vi "collsions_at_different_pressures.vi"() -> ()   [LabVIEW 2019]
uses:
  <instrlib>/niScope/Controls/niScope vertical coupling.ctl
  <instrlib>/niScope/Controls/niScope trigger source.ctl
  <instrlib>/niScope/Controls/niScope trigger coupling.ctl
  <instrlib>/niScope/Controls/niScope trigger slope.ctl
  <vilib>/Waveform/WDTFileIO.llb/Export Waveform To Spreadsheet File.vi
  <vilib>/Analysis/NI_AALBase.lvlib
panel:
  in  "Lower bound":dbl=4e-06
  in  "Step size":dbl=5e-07
  in  "Upper bound":dbl=5e-05
  in  "Channel":u16(ring) items=["1", "2"]
  in  "Eqilibration time / s":u32
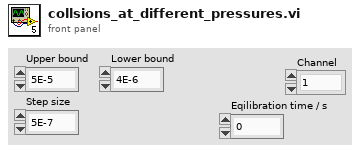
[diagram p1: front panel]
types:
  T1 = typedef "niScope vertical coupling.ctl" = i32
  T2 = typedef "niScope trigger source.ctl" = string
  T3 = typedef "niScope trigger coupling.ctl" = u16
  T4 = typedef "niScope trigger slope.ctl" = i32
  T5 = cluster{"C2 vertical offset":dbl, "C2 vertical range":dbl, "C2 probe attenuation":dbl, "C2 vertical coupling":T1, "C2 maximum input frequency":dbl, "C2 input impedance":u32, "C2 enabled":bool, "C1 input impedance":u32, "C1 maximum input frequency":dbl, "C1 enabled":bool, "C1 vertical offset":dbl, "C1 vertical range":dbl, "C1 probe attenuation":dbl, "C1 vertical coupling":T1, "Samples":i64, "tmax (\\mu s) ":dbl, "Trigger source":T2, "Trigger coupling":T3, "Trigger level":dbl, "Trigger slope":T4, "Trigger delay":dbl, "Enforce realtime":bool, "Aquisition Frequency / Hz":dbl, "Aqusition Time / ms":u32, "Scope Channel":refnum<k15>}
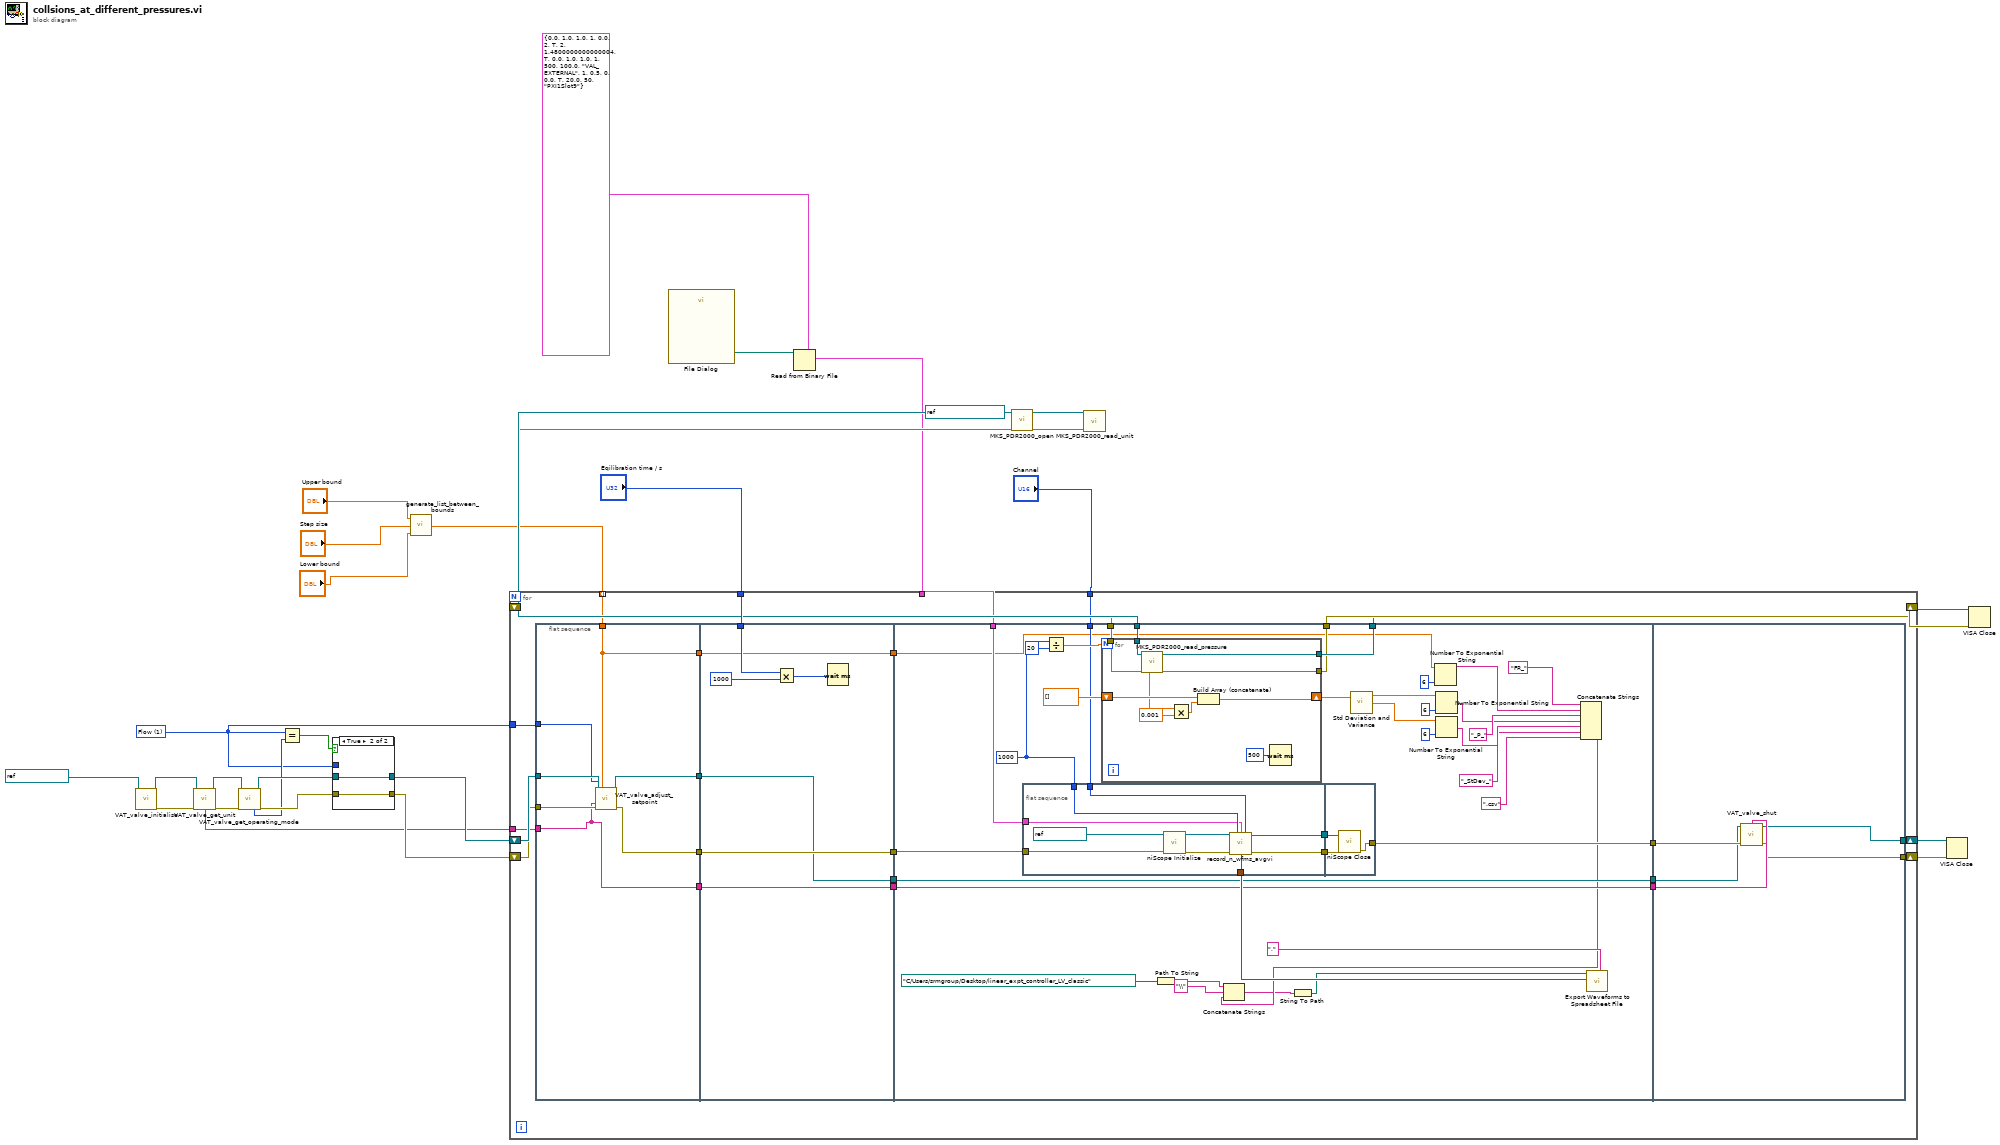
[diagram p0: block diagram]
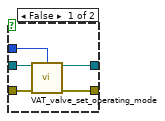
[diagram p2: hidden frame]
diagram:
  w19 = u16 1 items=["Pressure", "Flow", "Stop"] ("Operating Mode")
  n1 = call "VAT_valve_initialise.vi"("VAT Valve COM port"=refnum<visa-resource-name> "VAT_valve") -> ("VAT Valve COM port out"=w30:refnum<visa-resource-name>, "error out"=w29:errorcluster)  [unwired: 7 in, 6 out]
  n2 = call "VAT_valve_get_unit.vi"("VAT Valve COM port"=w30, "error in (no error)"=w29) -> ("VAT Valve COM port out"=w28:refnum<visa-resource-name>, "Unit"=w20:string, "error out"=w27:errorcluster)  [unwired: 11 in]
  n3 = call "VAT_valve_get_operating_mode.vi"("VAT Valve COM port"=w28, "error in (no error)"=w27) -> ("VAT Valve COM port out"=w26:refnum<visa-resource-name>, "Operating Mode"=w23:u16, "error out"=w25:errorcluster)  [unwired: 10 in, 1 out]
  n4 = Equal?(x=w19, y=w23) -> (x = y?=w24:bool)
  n5 = case shown="True" w24 {
    tunnel: w26 -> [w36 w38]
    tunnel: w25 -> [w35 w37]
    tunnel: [w34 w38] -> w22
    tunnel: [w33 w37] -> w21
    tunnel: w19 -> [w32 _]
    frame False {
      n6 = call "VAT_valve_set_operating_mode.vi"("VAT Valve COM port"=w36, "Operating Mode"=w32, "error in (no error)"=w35) -> ("VAT Valve COM port out"=w34:refnum<visa-resource-name>, "error out"=w33:errorcluster)  [unwired: 11 in]
    }
    frame True {
    }
  }
  n7 = call "generate_list_between_bounds.vi"("Upper bound"="Upper bound", "Step size"="Step size", "Lower bound"="Lower bound") -> ("Array"=w1:dbl[])  [unwired: 2 in]
  n8 = call "File Dialog"() -> ("selected path"=w9:path)  [unwired: 12 in, 3 out]
  n9 = Read from Binary File(5:T5 {"C2 vertical offset"=0.0, "C2 vertical range"=1.0, "C2 probe attenuation"=1.0, "C2 vertical coupling"=1, "C2 maximum input frequency"=0.0, "C2 input impedance"=2, "C2 enabled"=TRUE, "C1 input impedance"=2, "C1 maximum input frequency"=1.4800000000000004, "C1 enabled"=TRUE, "C1 vertical offset"=0.0, "C1 vertical range"=1.0, "C1 probe attenuation"=1.0, "C1 vertical coupling"=1, "Samples"=500, "tmax (\\mu s) "=100.0, "Trigger source"="VAL_EXTERNAL", "Trigger coupling"=1, "Trigger level"=0.5, "Trigger slope"=0, "Trigger delay"=0.0, "Enforce realtime"=TRUE, "Aquisition Frequency / Hz"=20.0, "Aqusition Time / ms"=50, "Scope Channel"="PXI1Slot9"} ("Cluster"), 11:w9) -> (2:w8:T5)  [unwired: 4 in, 3 out]
  n10 = call "MKS_PDR2000_open.vi"("PDR2000 COM port"=refnum<visa-resource-name> "PDR_2000") -> ("error out"=w15:errorcluster, "PDR2000 COM port out"=w16:refnum<visa-resource-name>)  [unwired: 9 in]
  n11 = call "MKS_PDR2000_read_unit.vi"("PDR2000 COM port"=w16, "error in (no error)"=w15) -> ("PDR2000 COM port out"=w14:refnum<visa-resource-name>, "error out"=w13:errorcluster)  [unwired: 11 in, 1 out]
  n12 = for {
    tunnel: w20 -> [w50]
    tunnel: w19 -> [w49]
    tunnel: "Eqilibration time / s" -> [w48]
    tunnel: w8 -> [w43]
    tunnel: "Channel" -> [w40]
    shift-right: [w42] -> w7
    shift-left: w22 -> [w52]
    shift-right: [w41] -> w6
    shift-left: w21 -> [w51]
    shift-right: [w44] -> w11
    shift-left: w14 -> [w47]
    shift-right: [w45] -> w12
    shift-left: w13 -> [w46]
    tunnel: w1 -> [w39] mode=indexing
    n13 = flat-sequence {
      tunnel: w52 -> [w70]
      tunnel: w51 -> [w69]
      tunnel: w50 -> [w65]
      tunnel: w39 -> [w64]
      tunnel: w49 -> [w68]
      tunnel: [w67] -> w63
      tunnel: [w66] -> w62
      tunnel: [w65] -> w61
      tunnel: [w64] -> w60
      tunnel: w48 -> [w76]
      tunnel: [w74] -> w59
      tunnel: w63 -> [w74]
      tunnel: [w73] -> w58
      tunnel: w62 -> [w73]
      tunnel: w61 -> [w72]
      tunnel: [w72] -> w57
      tunnel: [w71] -> w56
      tunnel: w60 -> [w71]
      tunnel: w47 -> [w115]
      tunnel: w46 -> [w114]
      tunnel: [w105] -> w45
      tunnel: [w113] -> w44
      tunnel: w59 -> [w111]
      tunnel: [w101] -> w55
      tunnel: w58 -> [w100]
      tunnel: [w100] -> w54
      tunnel: w43 -> [w99]
      tunnel: w57 -> [w98]
      tunnel: [w98] -> w53
      tunnel: w40 -> [w97]
      tunnel: w56 -> [w88]
      tunnel: w55 -> [w143]
      tunnel: w54 -> [w142]
      tunnel: w53 -> [w141]
      tunnel: [w140] -> w42
      tunnel: [w139] -> w41
      frame #0 {
        n14 = call "VAT_valve_adjust_setpoint.vi"("VAT Valve COM port"=w70, "Flow"=w64, "Operating Mode"=w68, "Unit"=w65, "error in (no error)"=w69) -> ("VAT Valve COM port out"=w66:refnum<visa-resource-name>, "error out"=w67:errorcluster)  [unwired: 9 in]
      }
      frame #1 {
        n15 = Multiply(x=w76, y=u32 1000 ("milliseconds to wait")) -> (x*y=w75:u32)
        n16 = Wait (ms)(milliseconds to wait=w75) -> ()  [unwired: 1 out]
      }
      frame #2 {
        w107 = 1000 ("Number of Sweeps")
        n17 = flat-sequence {
          tunnel: w111 -> [w132]
          tunnel: [w131] -> w110
          tunnel: [w130] -> w109
          tunnel: w107 -> [w129]
          tunnel: [w128] -> w102
          tunnel: w99 -> [w127]
          tunnel: w97 -> [w126]
          tunnel: w110 -> [w138]
          tunnel: w109 -> [w137]
          tunnel: [w136] -> w101
          frame #0 {
            n18 = call <instrlib>:"niScope Initialize.vi"("resource name"=refnum<k15> "PXI1Slot9" ("instrument handle"), "error in"=w132) -> ("instrument handle"=w135:refnum<k15>, "error out"=w134:errorcluster)  [unwired: 12 in]
            n19 = call "record_n_wfms_avgvi.vi"("instrument handle"=w135, "Number of Sweeps"=w129, "Scope Config Data"=w127, "Channel"=w126, "Error in (no error)"=w134) -> ("instrument handle out"=w131:refnum<k15>, "Waveform"=w128:waveform(dbl), "Error out"=w130:errorcluster)  [unwired: 8 in]
          }
          frame #1 {
            n20 = call <instrlib>:"niScope Close.vi"("instrument handle"=w138, "error in"=w137) -> ("error out"=w136:errorcluster)  [unwired: 13 in]
          }
        }
        n21 = Divide(x=w107, y=20) -> (x/y=w108:dbl)
        n22 = for {
          N: w108 -> [_]
          tunnel: w115 -> [w125]
          tunnel: w114 -> [w124]
          tunnel: [w123] -> w113
          tunnel: [w122] -> w105
          shift-right: [w120] -> w104
          shift-left: dbl[] [] -> [w121]
          n23 = call "MKS_PDR2000_read_pressure.vi"("error in (no error)"=w124, "PDR2000 COM port"=w125) -> ("error out"=w122:errorcluster, "PDR2000 COM port out"=w123:refnum<visa-resource-name>, "Channel 1 Pressure"=w118:dbl)  [unwired: 6 in, 1 out]
          n24 = Multiply(x=w118, y=0.001) -> (x*y=w119:dbl)
          n25 = Build Array (concatenate)(w121, w119) -> (w120:dbl[])
          n26 = Wait (ms)(milliseconds to wait=u32 500) -> ()  [unwired: 1 out]
        }
        n27 = Path To String(path=path "C:/Users/srmgroup/Desktop/linear_expt_controller_LV_classic" ("file path (dialog if empty)")) -> (string=w82:string)
        n28 = call <vilib>:"Std Deviation and Variance.vi"("X"=w104) -> ("mean"=w96:dbl, "standard deviation"=w95:dbl)  [unwired: 1 in, 1 out]
        n29 = Number To Exponential String(number=w88, precision (6)=i16 6) -> (E-format string=w86:string)  [unwired: 2 in]
        n30 = Number To Exponential String(number=w96, precision (6)=i16 6) -> (E-format string=w85:string)  [unwired: 2 in]
        n31 = Number To Exponential String(number=w95, precision (6)=i16 6) -> (E-format string=w84:string)  [unwired: 2 in]
        n32 = Concatenate Strings("FR_" ("string"), w86, "_P_" ("string"), w85, "_StDev_" ("string"), w84, ".csv" ("string")) -> (w80:string)
        n33 = Concatenate Strings(w82, "\\" ("element"), w80) -> (w79:string)
        n34 = String To Path(string=w79) -> (path=w78:path)
        n35 = call-poly <vilib>:"Export Waveforms to Spreadsheet File.vi"("delimiter (Tab)"=",", "waveform"=w102, "file path (dialog if empty)"=w78) -> ()  [unwired: 7 in, 2 out]
      }
      frame #3 {
        n36 = call "VAT_valve_shut.vi"("VAT Valve COM port"=w142, "Unit"=w141, "error in (no error)"=w143) -> ("VAT Valve COM port out"=w140:refnum<visa-resource-name>, "error out"=w139:errorcluster)  [unwired: 10 in, 1 out]
      }
    }
  }
  n37 = VISA Close(VISA resource name=w7, error in (no error)=w6) -> ()  [unwired: 1 out]
  n38 = VISA Close(VISA resource name=w11, error in (no error)=w12) -> ()  [unwired: 1 out]
